vi "simple_insert_example.vi"() -> ()   [LabVIEW 2020, in "Data.PG.lvclass"]
uses:
  Data.PG.lvclass
panel:
  in  "path":string
  in  "milliseconds to wait between points":u32
  in  "How many points":i32
  in  "Data.PG in":refnum<class "Data.PG.lvclass">
  out "Data.PG out":refnum<class "Data.PG.lvclass">
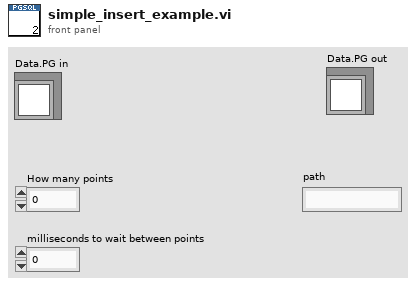
[diagram p1: front panel]
types:
  T1 = cluster{"host":string, "port":string, "user":string, "dbname":string, "password":string}
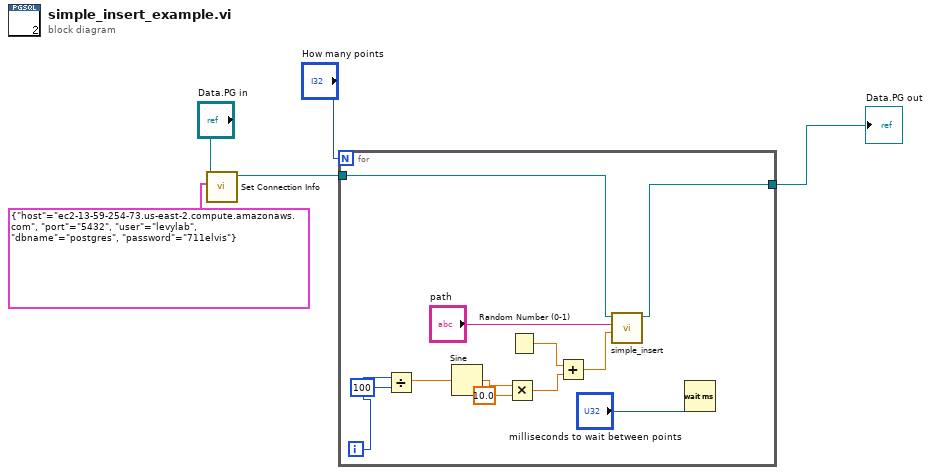
[diagram p0: block diagram]
diagram:
  n1 = call "Set Connection Info.vi"("connection info"=T1 {"host"="ec2-13-59-254-73.us-east-2.compute.amazonaws.com", "port"="5432", "user"="levylab", "dbname"="postgres", "password"="711elvis"}, "Data.PG in"="Data.PG in") -> ("Data.PG out"=w3:refnum<class "Data.PG.lvclass">)  [unwired: 8 in, 1 out]
  n2 = for {
    N: "How many points" -> [_]
    tunnel: w3 -> [w10]
    tunnel: [w9] -> w2
    i -> [w16]
    n3 = Divide(x=w16, y=100) -> (x/y=w17:dbl)
    n4 = Sine(x=w17) -> (sin(x)=w14:dbl)
    n5 = Multiply(x=w14, y=10.0) -> (x*y=w12:dbl)
    n6 = Random Number (0-1)() -> (number: 0 to 1=w11:dbl)
    n7 = Add(x=w11, y=w12) -> (x+y=w8:dbl)
    n8 = call "simple_insert.vi"("Value"=w8, "path table:column"="path", "Data.PG in"=w10) -> ("Data.PG out"=w9:refnum<class "Data.PG.lvclass">)  [unwired: 7 in, 1 out]
    n9 = Wait (ms)(milliseconds to wait="milliseconds to wait between points") -> ()  [unwired: 1 out]
  }
  "Data.PG out" <- w2
